vi "总磷总氮通讯.vi"() -> ()   [LabVIEW 2016, in "斯坦道总磷总氮.lvlib"]
uses:
  <vilib>/NI/Modbus Library/API/Wrapper/Create TCP Slave.vi
  <vilib>/Utility/config.llb/Write Key (Boolean).vi
  <vilib>/Utility/config.llb/Write Key (String).vi
  <vilib>/Plasmionique/MB Master/MB_Master/MB_Master.lvclass
  <vilib>/NI/Modbus Library/API/slave/Modbus Slave.lvclass
  <vilib>/Utility/config.llb/NI_LVConfig.lvlib
  <vilib>/Plasmionique/MB Master/MB Master.lvlib
  <vilib>/NI/Modbus Library/API/Wrapper/API Main.lvlib
panel:
  out "总氮测量数据区":u16[](array[numeric])
  out "总氮状态告警区":u16[](array[numeric])
  out "总磷状态告警区":u16[](array[numeric])
  out "总磷测量数据区":u16[](array[numeric])
  out "序列号":string
  out "状态告警区":T1 {"告警代码" items=["无告警", "缺试剂告警", "缺水样告警", "缺蒸馏水告警", "缺标液告警", "仪表漏液告警", "标定异常告警", "超量程告警", "加热异常", "低试剂预警", "超上限告警", "超下限告警", "仪表内部其他异常", "滴定异常告警", "电极异常告警", "量程切换告警", "参数设置告警", "PH电极电位异常", "电导率电极异常", "浊度光度异常", "溶解氧电极异常", "溶解氧光强异常", "温度异常告警", "PH异常告警", "溶解氧异常告警", "电导率异常告警", "浊度异常告警", "叶绿素异常告警", "藻密度异常告警", "蓝绿藻异常告警", "ORP异常告警", "氨氮异常告警", "清洁刷异常告警", "SD卡异常告警", "蓝牙异常告警", "Wifi异常告警", "流程异常告警"]; "故障代码" items=["无故障", "电机故障", "温度故障", "通讯故障", "滴定故障"]}
  out "测量数据区":T2 {"单位" items=["ug/L", "mg/L", "ppm", "mg/m3", "cm", "ppb", "ug/m3", "%", "nmol/mol", "umol/mol", "MPN/L", "MPN/100ml", "ng/m3", "NTU", "无量纲", "ms/cm", "us/cm", "℃", "mV", "万个/L"]}
  out "status":bool
  out "关键参数区":T3
  in  "读关键参数区":bool
  in  "读状态告警区":bool
  in  "读测量数据区":bool
  in  "站号":u16(ring) items=["总磷"=1, "氨氮"=3]
  in  "停止":bool
  in  "启动":bool
  in  "控制命令":u16(ring) items=["启动测量"=1, "标样核查"=2, "零点核查"=3, "跨度核查"=4, "空白测试"=5, "平行样测试"=6, "加标回收"=7, "空白校准"=8, "标样校准"=9, "初始化（清洗）"=10, "停止测试"=11, "仪器重启"=12, "校时"=13, "模式设置"=14, "测量间隔设置"=15]
  in  "控制命令参数":u16[](array[numeric]) format="%04xH"
  in  "VISA Resource":refnum<visa-resource-name>
  in  "启用模块":bool
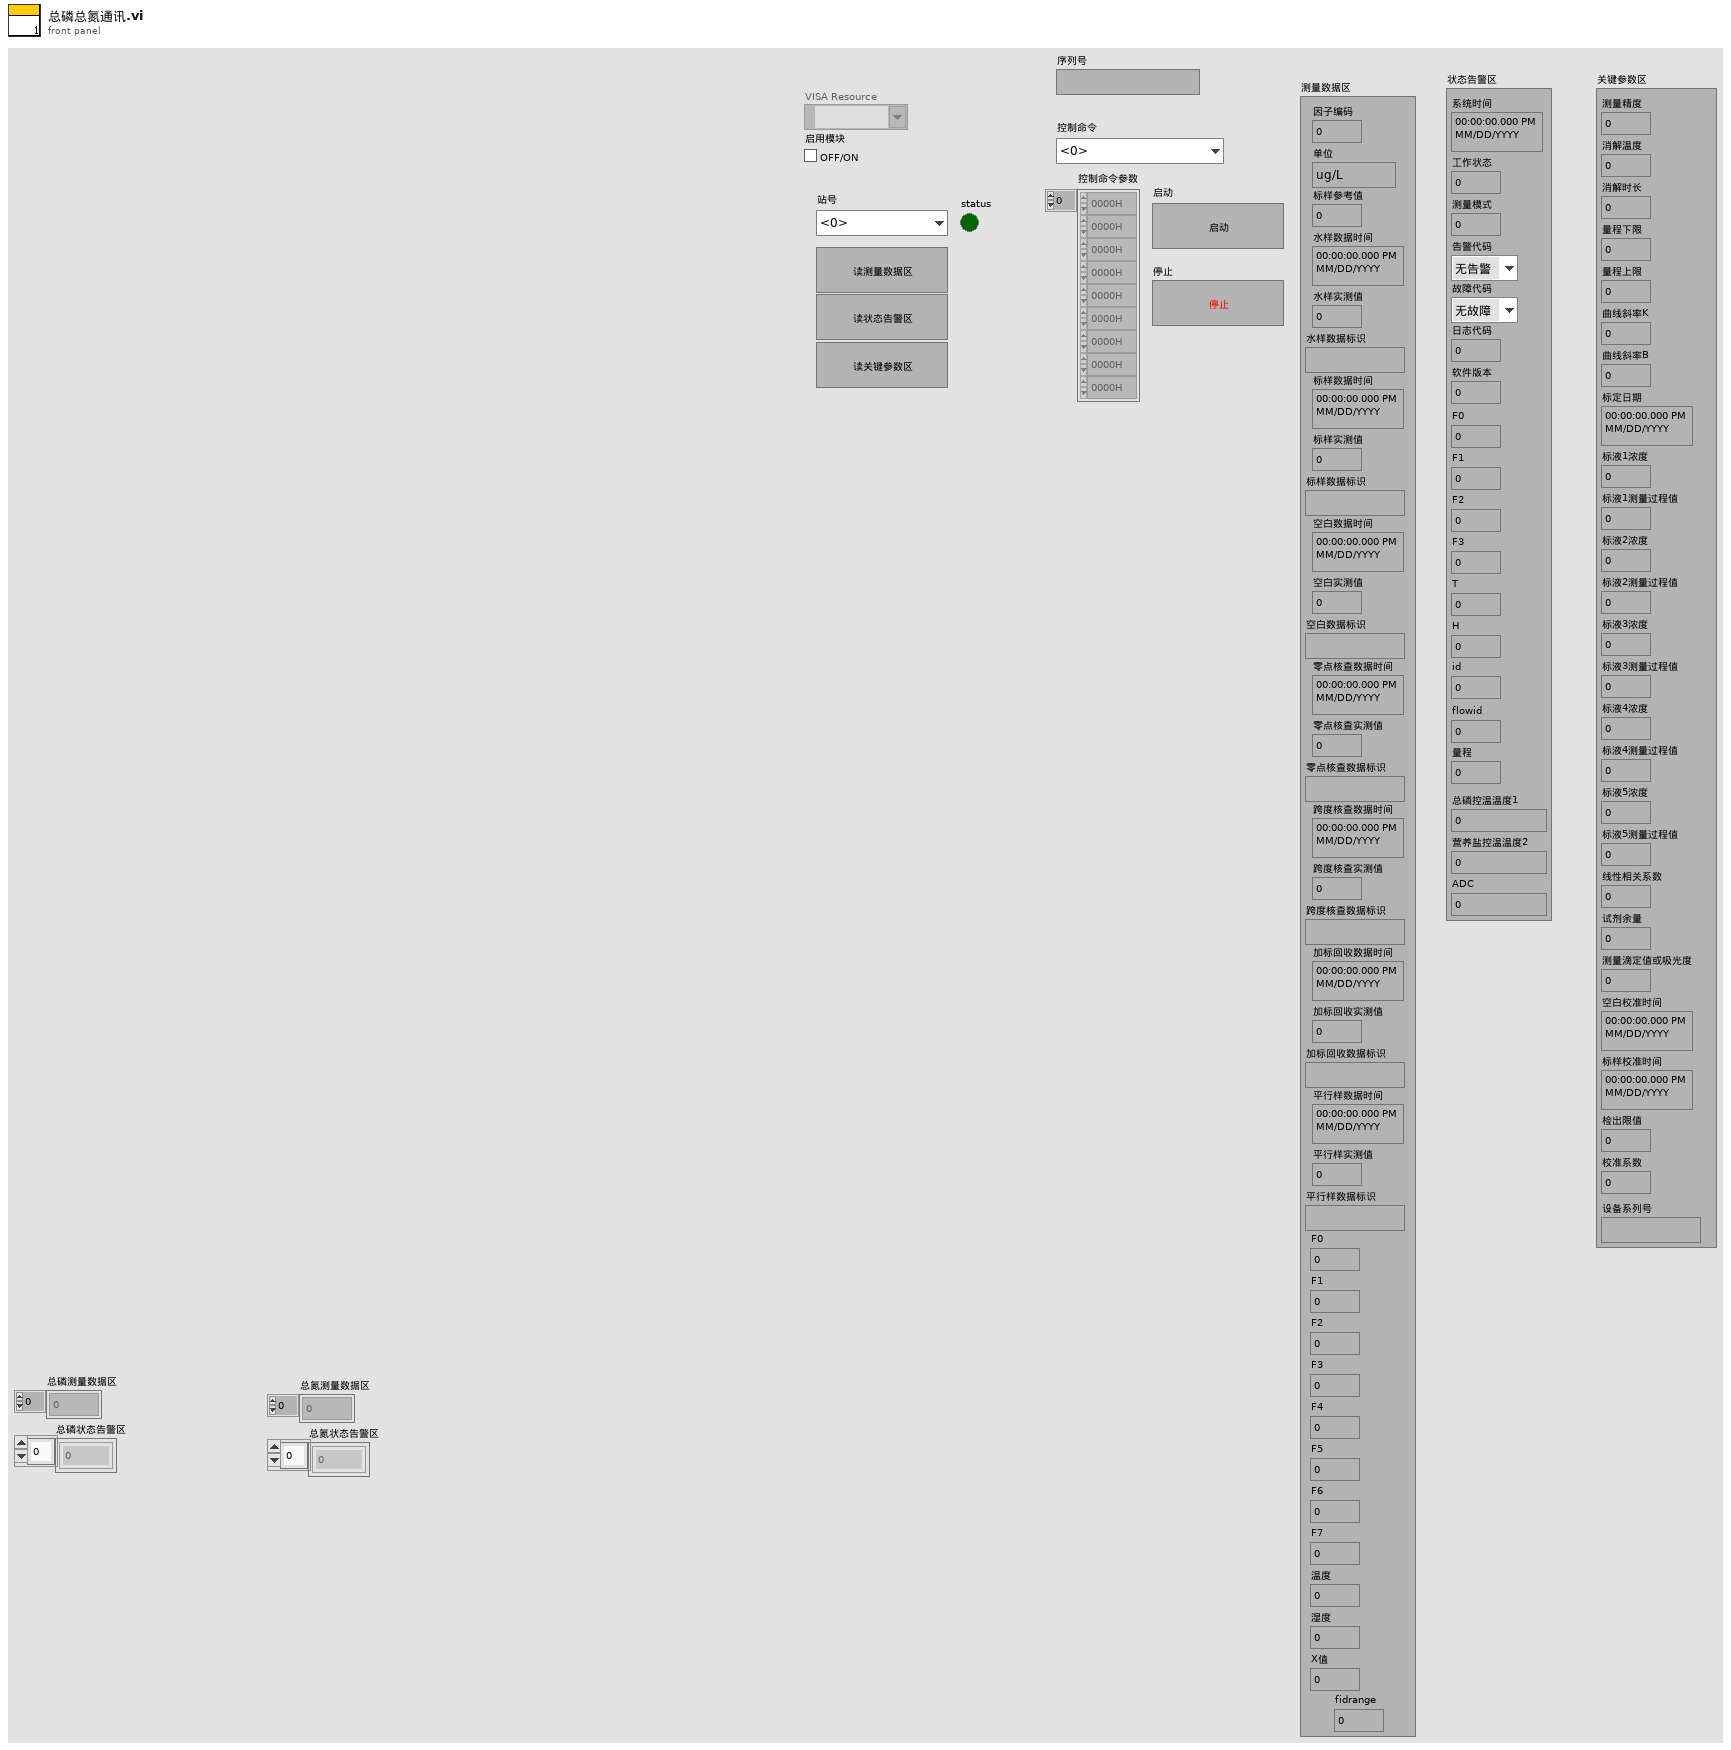
[diagram p1: front panel]
types:
  T1 = cluster{"系统时间":timestamp, "工作状态":u16, "测量模式":u16, "告警代码":u16, "故障代码":u16, "日志代码":u16, "软件版本":u16, "F0":sgl, "F1":sgl, "F2":sgl, "F3":sgl, "T":sgl, "H":sgl, "id":u16, "flowid":u16, "量程":u16, "总磷控温温度1":sgl, "营养盐控温温度2":sgl, "ADC":sgl}
  T2 = cluster{"因子编码":u32, "单位":u16, "标样参考值":sgl, "水样数据时间":timestamp, "水样实测值":sgl, "水样数据标识":string, "标样数据时间":timestamp, "标样实测值":sgl, "标样数据标识":string, "空白数据时间":timestamp, "空白实测值":sgl, "空白数据标识":string, "零点核查数据时间":timestamp, "零点核查实测值":sgl, "零点核查数据标识":string, "跨度核查数据时间":timestamp, "跨度核查实测值":sgl, "跨度核查数据标识":string, "加标回收数据时间":timestamp, "加标回收实测值":sgl, "加标回收数据标识":string, "平行样数据时间":timestamp, "平行样实测值":sgl, "平行样数据标识":string, "F0":sgl, "F1":sgl, "F2":sgl, "F3":sgl, "F4":sgl, "F5":sgl, "F6":sgl, "F7":sgl, "温度":sgl, "湿度":sgl, "X值":sgl, "fidrange":u16}
  T3 = cluster{"测量精度":u16, "消解温度":u16, "消解时长":u16, "量程下限":sgl, "量程上限":sgl, "曲线斜率K":sgl, "曲线斜率B":sgl, "标定日期":timestamp, "标液1浓度":sgl, "标液1测量过程值":sgl, "标液2浓度":sgl, "标液2测量过程值":sgl, "标液3浓度":sgl, "标液3测量过程值":sgl, "标液4浓度":sgl, "标液4测量过程值":sgl, "标液5浓度":sgl, "标液5测量过程值":sgl, "线性相关系数":sgl, "试剂余量":u32, "测量滴定值或吸光度":sgl, "空白校准时间":timestamp, "标样校准时间":timestamp, "检出限值":sgl, "校准系数":sgl, "设备系列号":string}
  T4 = typedef "NI_LVConfig.lvlib/Config Data RefNum.ctl" = refnum<k1>
  T5 = enum8{"Enabled", "Disabled", "Disabled and Grayed Out"}
  T6 = cluster{"系统时间":timestamp, "工作状态":enum16{"空闲", "水样测试", "标样核查", "零点核查", "跨度核查", "空白测试", "平行样测试", "加标回收", "空白校准", "标样校准", "初始化（清洗）"}, "测量模式":enum16{"待机", "连续模式", "周期模式", "定点模式", "受控模式", "手动模式"}, "告警代码":u16, "故障代码":u16, "日志代码":u16, "软件版本":u16, "F0":sgl, "F1":sgl, "F2":sgl, "F3":sgl, "T":sgl, "H":sgl, "id":u16, "flowid":u16, "量程":u16, "总磷控温温度1":sgl, "营养盐控温温度2":sgl, "ADC":sgl}
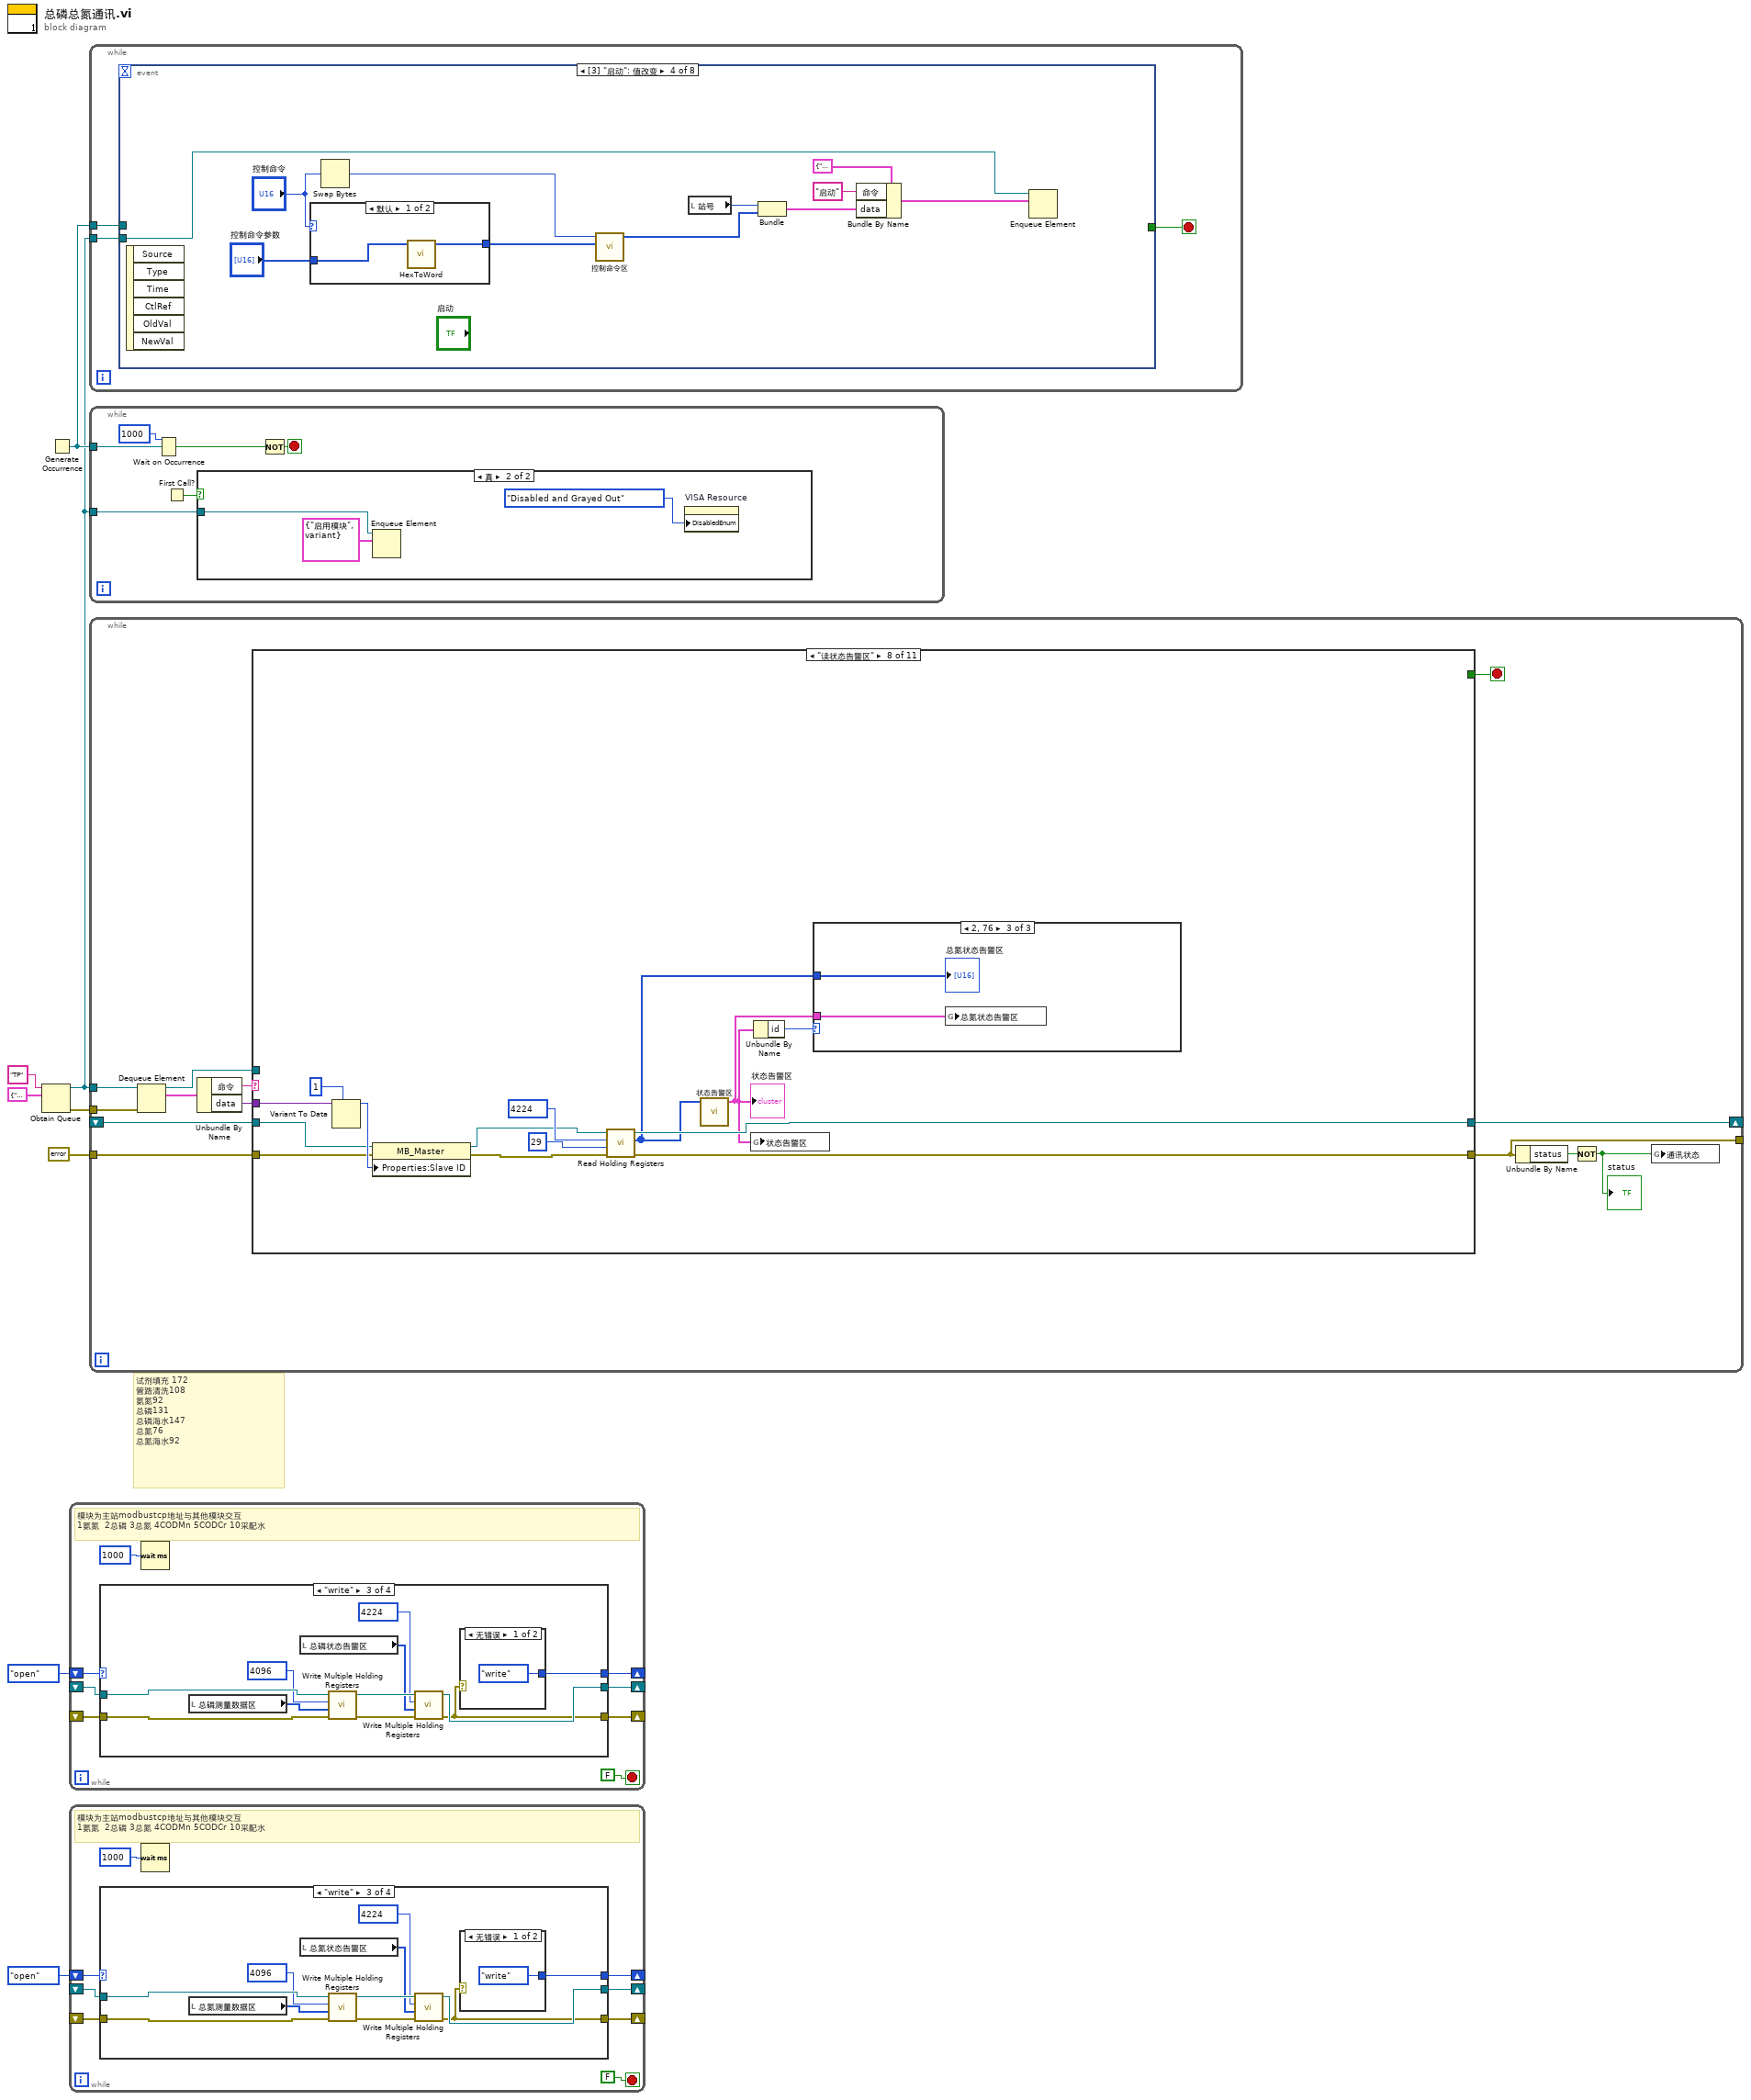
[diagram p0: block diagram]
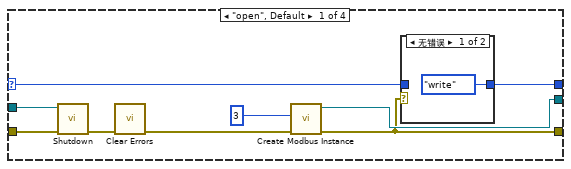
[diagram p2: hidden frame]
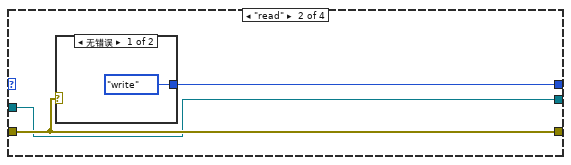
[diagram p4: hidden frame]
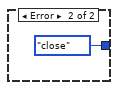
[diagram p5: hidden frame]
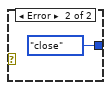
[diagram p6: hidden frame]
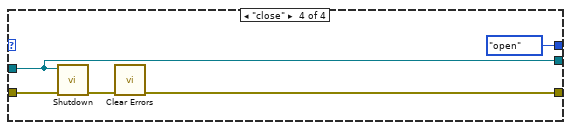
[diagram p7: hidden frame]
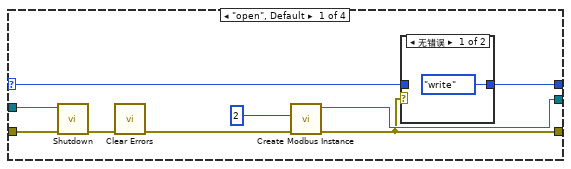
[diagram p8: hidden frame]
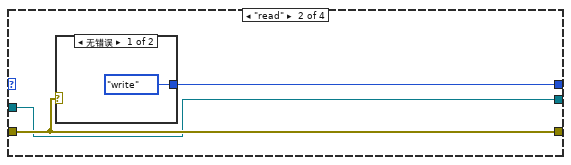
[diagram p10: hidden frame]
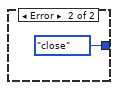
[diagram p11: hidden frame]
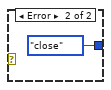
[diagram p12: hidden frame]
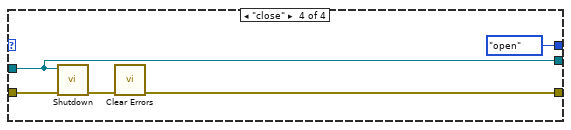
[diagram p13: hidden frame]
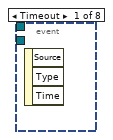
[diagram p15: hidden frame]
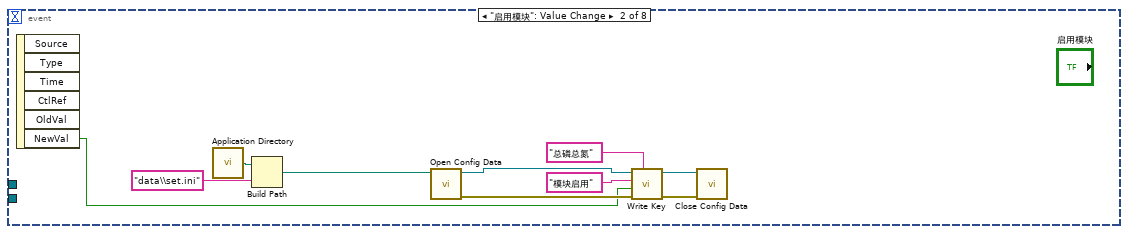
[diagram p16: hidden frame]
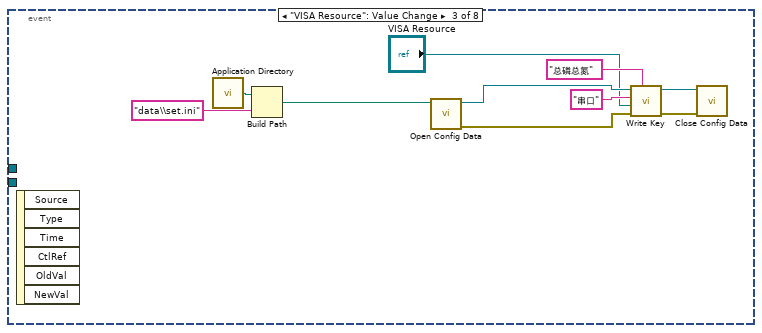
[diagram p17: hidden frame]
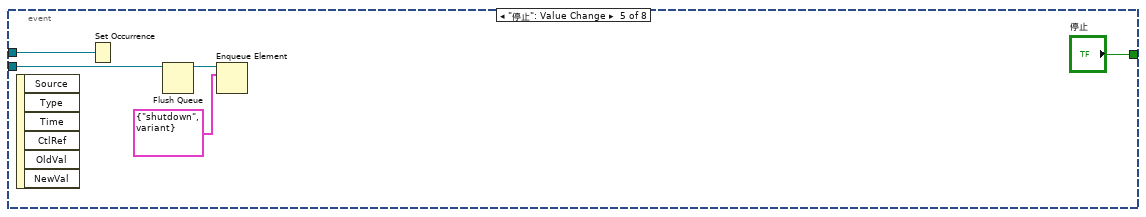
[diagram p19: hidden frame]
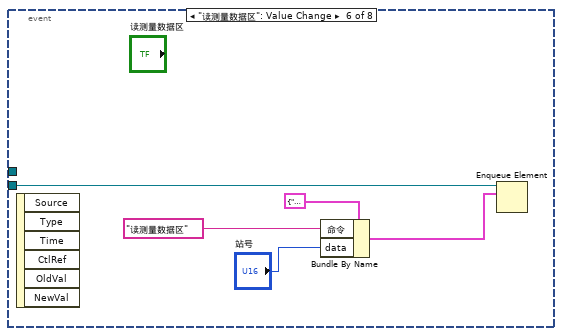
[diagram p20: hidden frame]
diagram:
  # "试剂填充 172 \n管路清洗108\n氨氮92\n总磷131\n总磷海水147\n总氮76\n总氮海水92"
  n1 = Obtain Queue(name (unnamed)="TP" ("名称（未命名）"), element data type=cluster{"命令":string, "data":variant} {"命令"="", "data"=variant}) -> (queue out=w3:refnum<queue>, error out=w6:errorcluster)  [unwired: 3 in, 1 out]
  n2 = Generate Occurrence() -> (w4:refnum<k4>)
  n3 = while {
    shift-right: [w14] -> _
    shift-left: _ -> [w16]
    shift-right: [w13] -> _
    shift-left: _ -> [w15]
    shift-right: [w10] -> _
    shift-left: enum16{"open", "read", "write", "close"}."open" -> [w11]
    stop <- FALSE stop-if-true
    # "模块为主站modbustcp地址与其他模块交互\n1氨氮  2总磷 3总氮 4CODMn 5CODCr 10采配水"
    n4 = case shown="\"write\"" w11 {
      selector: w11 -> [w25 _ _ _]
      tunnel: w16 -> [w19 w28 w42 w48]
      tunnel: w15 -> [w18 w29 w41 w47]
      tunnel: [w22 w28 w37 w48] -> w14
      tunnel: [w21 w29 w36 w50] -> w13
      tunnel: [w24 w30 w43 enum16{"open", "read", "write", "close"}."open"] -> w10
      frame "open", Default {
        n5 = call-dynamic "Shutdown.vi"("error in"=w18, "Modbus slave in"=w19) -> ("error out"=w17:errorcluster)  [unwired: 9 in]
        n6 = call <vilib>:"Clear Errors.vi"("error in (no error)"=w17) -> ("error out"=w20:errorcluster)  [unwired: 5 in, 1 out]
        n7 = call-poly <vilib>:"Create Modbus Instance.vi"("error in"=w20, "port (502)"=u16 2) -> ("error out"=w21:errorcluster, "TCP slave instance"=w22:refnum<class "Modbus Slave.lvclass">)  [unwired: 8 in]
        n8 = case shown="无错误" w21 {
          tunnel: w25 -> [_ w27]
          tunnel: [enum16{"open", "read", "write", "close"}."write" w27] -> w24
          frame No Error {
          }
          frame Error {
          }
        }
      }
      frame "read" {
        n9 = case shown="无错误" w29 {
          tunnel: [enum16{"open", "read", "write", "close"}."write" enum16{"open", "read", "write", "close"}."close"] -> w30
          frame No Error {
          }
          frame Error {
          }
        }
      }
      frame "write" {
        n10 = local read "总磷测量数据区"() -> (w35:u16[])
        n11 = local read "总磷状态告警区"() -> (w33:u16[])
        n12 = call-dynamic "Write Multiple Holding Registers.vi"("error in"=w41, "registers to write"=w35, "starting address"=u16 4096, "Modbus slave in"=w42) -> ("error out"=w38:errorcluster, "Modbus slave out"=w39:refnum<class "Modbus Slave.lvclass">)  [unwired: 6 in]
        n13 = call-dynamic "Write Multiple Holding Registers.vi"("error in"=w38, "registers to write"=w33, "starting address"=u16 4224, "Modbus slave in"=w39) -> ("error out"=w36:errorcluster, "Modbus slave out"=w37:refnum<class "Modbus Slave.lvclass">)  [unwired: 6 in]
        n14 = case shown="无错误" w36 {
          tunnel: [enum16{"open", "read", "write", "close"}."write" enum16{"open", "read", "write", "close"}."close"] -> w43
          frame No Error {
          }
          frame Error {
          }
        }
      }
      frame "close" {
        n15 = call-dynamic "Shutdown.vi"("error in"=w47, "Modbus slave in"=w48) -> ("error out"=w46:errorcluster)  [unwired: 9 in]
        n16 = call <vilib>:"Clear Errors.vi"("error in (no error)"=w46) -> ("error out"=w50:errorcluster)  [unwired: 5 in, 1 out]
      }
    }
    n17 = Wait (ms)(milliseconds to wait=u32 1000 ("等待时间（毫秒）")) -> ()  [unwired: 1 out]
  }
  n18 = while {
    shift-right: [w56] -> _
    shift-left: _ -> [w58]
    shift-right: [w55] -> _
    shift-left: _ -> [w57]
    shift-right: [w52] -> _
    shift-left: enum16{"open", "read", "write", "close"}."open" -> [w53]
    stop <- FALSE stop-if-true
    # "模块为主站modbustcp地址与其他模块交互\n1氨氮  2总磷 3总氮 4CODMn 5CODCr 10采配水"
    n19 = case shown="\"write\"" w53 {
      selector: w53 -> [w67 _ _ _]
      tunnel: w58 -> [w61 w70 w84 w90]
      tunnel: w57 -> [w60 w71 w83 w89]
      tunnel: [w64 w70 w79 w90] -> w56
      tunnel: [w63 w71 w78 w92] -> w55
      tunnel: [w66 w72 w85 enum16{"open", "read", "write", "close"}."open"] -> w52
      frame "open", Default {
        n20 = call-dynamic "Shutdown.vi"("error in"=w60, "Modbus slave in"=w61) -> ("error out"=w59:errorcluster)  [unwired: 9 in]
        n21 = call <vilib>:"Clear Errors.vi"("error in (no error)"=w59) -> ("error out"=w62:errorcluster)  [unwired: 5 in, 1 out]
        n22 = call-poly <vilib>:"Create Modbus Instance.vi"("error in"=w62, "port (502)"=u16 3) -> ("error out"=w63:errorcluster, "TCP slave instance"=w64:refnum<class "Modbus Slave.lvclass">)  [unwired: 8 in]
        n23 = case shown="无错误" w63 {
          tunnel: w67 -> [_ w69]
          tunnel: [enum16{"open", "read", "write", "close"}."write" w69] -> w66
          frame No Error {
          }
          frame Error {
          }
        }
      }
      frame "read" {
        n24 = case shown="无错误" w71 {
          tunnel: [enum16{"open", "read", "write", "close"}."write" enum16{"open", "read", "write", "close"}."close"] -> w72
          frame No Error {
          }
          frame Error {
          }
        }
      }
      frame "write" {
        n25 = local read "总氮测量数据区"() -> (w77:u16[])
        n26 = local read "总氮状态告警区"() -> (w75:u16[])
        n27 = call-dynamic "Write Multiple Holding Registers.vi"("error in"=w83, "registers to write"=w77, "starting address"=u16 4096, "Modbus slave in"=w84) -> ("error out"=w80:errorcluster, "Modbus slave out"=w81:refnum<class "Modbus Slave.lvclass">)  [unwired: 6 in]
        n28 = call-dynamic "Write Multiple Holding Registers.vi"("error in"=w80, "registers to write"=w75, "starting address"=u16 4224, "Modbus slave in"=w81) -> ("error out"=w78:errorcluster, "Modbus slave out"=w79:refnum<class "Modbus Slave.lvclass">)  [unwired: 6 in]
        n29 = case shown="无错误" w78 {
          tunnel: [enum16{"open", "read", "write", "close"}."write" enum16{"open", "read", "write", "close"}."close"] -> w85
          frame No Error {
          }
          frame Error {
          }
        }
      }
      frame "close" {
        n30 = call-dynamic "Shutdown.vi"("error in"=w89, "Modbus slave in"=w90) -> ("error out"=w88:errorcluster)  [unwired: 9 in]
        n31 = call <vilib>:"Clear Errors.vi"("error in (no error)"=w88) -> ("error out"=w92:errorcluster)  [unwired: 5 in, 1 out]
      }
    }
    n32 = Wait (ms)(milliseconds to wait=u32 1000 ("等待时间（毫秒）")) -> ()  [unwired: 1 out]
  }
  n33 = while {
    tunnel: w3 -> [w95]
    tunnel: w4 -> [w93]
    stop <- w94 stop-if-true
    n34 = event shown="[3] \"启动\": 值改变" {
      selector: _ -> [_ _ _ _ _ _ _ _]
      dyn-events: _ -> [_ _ _ _ _ _ _ _]
      timeout: _ -> [_ _ _ _ _ _ _ _]
      tunnel: w95 -> [_ _ _ w126 w133 w139 w144 w149]
      tunnel: [_ _ _ _ "停止" _ _ _] -> w94
      tunnel: w93 -> [_ _ _ _ w130 _ _ _]
      event Timeout {
        n35 = event-data() -> ()  [unwired: 1 in, 3 out]
      }
      event "启用模块": Value Change {
        n36 = event-data() -> ("NewVal"=w96:bool)  [unwired: 1 in, 5 out]
        n37 = call <vilib>:"Application Directory.vi"() -> ("Application Directory"=w98:path)
        n38 = Build Path(base path=w98, name or relative path="data\\set.ini" ("名称或相对路径")) -> (appended path=w99:path)
        n39 = call <vilib>:"Open Config Data.vi"("configuration file path"=w99) -> ("error out"=w105:errorcluster, "refnum"=w104:T4)  [unwired: 8 in, 1 out]
        n40 = call-poly <vilib>:"Write Key.vi"("section"="总磷总氮", "error in (no error)"=w105, "value"=w96, "key"="模块启用", "refnum"=w104) -> ("error out"=w101:errorcluster, "refnum out"=w97:T4)  [unwired: 4 in, 1 out]
        n41 = call <vilib>:"Close Config Data.vi"("error in (no error)"=w101, "refnum"=w97) -> ()  [unwired: 8 in, 2 out]
      }
      event "VISA Resource": Value Change {
        n42 = event-data() -> ()  [unwired: 1 in, 6 out]
        n43 = call <vilib>:"Application Directory.vi"() -> ("Application Directory"=w108:path)
        n44 = Build Path(base path=w108, name or relative path="data\\set.ini" ("名称或相对路径")) -> (appended path=w109:path)
        n45 = call <vilib>:"Open Config Data.vi"("configuration file path"=w109) -> ("error out"=w115:errorcluster, "refnum"=w114:T4)  [unwired: 8 in, 1 out]
        n46 = call-poly <vilib>:"Write Key.vi"("section"="总磷总氮", "error in (no error)"=w115, "value"="VISA Resource", "key"="串口", "refnum"=w114) -> ("error out"=w111:errorcluster, "refnum out"=w107:T4)  [unwired: 4 in, 1 out]
        n47 = call <vilib>:"Close Config Data.vi"("error in (no error)"=w111, "refnum"=w107) -> ()  [unwired: 8 in, 2 out]
      }
      event "启动": Value Change {
        n48 = event-data() -> ()  [unwired: 1 in, 6 out]
        n49 = case shown="默认" "控制命令" {
          tunnel: "控制命令参数" -> [w128 w129]
          tunnel: [w127 w129] -> w116
          frame Default {
            n50 = call "HexToWord.vi"("数组"=w128) -> ("WORD"=w127:u16[])  [unwired: 10 in]
          }
          frame 13 {
          }
        }
        n51 = Swap Bytes(anything="控制命令") -> (byte swapped=w119:u16)
        n52 = call "控制命令区.vi"("控制命令参数"=w116, "控制命令"=w119) -> ("控制命令"=w122:u16[])  [unwired: 9 in]
        n53 = local read "站号"() -> (w121:u16)
        n54 = Bundle("站号"=w121, "控制命令"=w122) -> (w120:cluster{"站号":u16, "控制命令":u16[]})  [unwired: 1 in]
        n55 = Bundle By Name(cluster=cluster{"命令":string, "data":variant} {"命令"="", "data"=variant} ("元素"), "命令"="启动", "data"=w120) -> (w124:cluster{"命令":string, "data":variant})
        n56 = Enqueue Element(queue=w126, element=w124) -> ()  [unwired: 2 in, 3 out]
      }
      event "停止": Value Change {
        n57 = event-data() -> ()  [unwired: 1 in, 6 out]
        n58 = Set Occurrence(w130) -> ()
        n59 = Flush Queue(queue=w133) -> (queue out=w132:refnum<queue>)  [unwired: 1 in, 2 out]
        n60 = Enqueue Element(queue=w132, element=cluster{"命令":string, "data":variant} {"命令"="shutdown", "data"=variant} ("元素")) -> ()  [unwired: 2 in, 3 out]
      }
      event "读测量数据区": Value Change {
        n61 = event-data() -> ()  [unwired: 1 in, 6 out]
        n62 = Bundle By Name(cluster=cluster{"命令":string, "data":variant} {"命令"="", "data"=variant} ("元素"), "命令"="读测量数据区", "data"="站号") -> (w137:cluster{"命令":string, "data":variant})
        n63 = Enqueue Element(queue=w139, element=w137) -> ()  [unwired: 2 in, 3 out]
      }
      event "读状态告警区": Value Change {
        n64 = event-data() -> ()  [unwired: 1 in, 6 out]
        n65 = local read "站号"() -> (w140:u16)
        n66 = Bundle By Name(cluster=cluster{"命令":string, "data":variant} {"命令"="", "data"=variant} ("元素"), "命令"="读状态告警区", "data"=w140) -> (w142:cluster{"命令":string, "data":variant})
        n67 = Enqueue Element(queue=w144, element=w142) -> ()  [unwired: 2 in, 3 out]
      }
      event "读关键参数区": Value Change {
        n68 = event-data() -> ()  [unwired: 1 in, 6 out]
        n69 = local read "站号"() -> (w145:u16)
        n70 = Bundle By Name(cluster=cluster{"命令":string, "data":variant} {"命令"="", "data"=variant} ("元素"), "命令"="读关键参数区", "data"=w145) -> (w147:cluster{"命令":string, "data":variant})
        n71 = Enqueue Element(queue=w149, element=w147) -> ()  [unwired: 2 in, 3 out]
      }
    }
  }
  n72 = while {
    tunnel: w4 -> [w155]
    tunnel: w3 -> [w151]
    stop <- w152 stop-if-true
    n73 = Wait on Occurrence(2:w155, 3:1000 ("毫秒超时(-1)")) -> (0:w153:bool)  [unwired: 1 in]
    n74 = First Call?() -> (First Call?: T/F=w150:bool)
    n75 = case shown="真" w150 {
      tunnel: w151 -> [_ w157]
      frame False {
      }
      frame True {
        n76 = Enqueue Element(queue=w157, element=cluster{"命令":string, "data":variant} {"命令"="启用模块", "data"=variant} ("元素")) -> ()  [unwired: 2 in, 3 out]
        n77 = property on="VISA Resource" class="VISAName"("DisabledEnum"=T5."Disabled and Grayed Out" ("禁用")) -> ()  [unwired: 2 in, 2 out]
      }
    }
    n78 = Not(x=w153) -> (.not. x?=w152:bool)
  }
  n79 = while {
    tunnel: w3 -> [w171]
    tunnel: w6 -> [w170]
    shift-right: [w168] -> _
    shift-left: _ -> [w167]
    tunnel: errorcluster {"status"=FALSE, "code"=0, "source"=""} ("error out") -> [w166]
    tunnel: [w161] -> _
    stop <- w169 stop-if-true
    n80 = Dequeue Element(queue=w171, error in (no error)=w170) -> (queue out=w162:refnum<queue>, element=w164:cluster{"命令":string, "data":variant})  [unwired: 1 in, 2 out]
    n81 = Unbundle By Name(w164) -> ("命令"=w165:string, "data"=w163:variant)
    n82 = case shown="\"读状态告警区\"" w165 {
      tunnel: w163 -> [_ _ _ w190 w201 w218 w228 w261 w279 w293 _]
      tunnel: w162 -> [_ _ _ _ _ _ _ _ _ _ w306]
      tunnel: [_ _ _ _ _ _ _ _ _ _ TRUE] -> w169
      tunnel: [w172 w174 w177 w193 w204 w220 w232 w270 w286 w300 w302] -> w168
      tunnel: [w173 w175 w178 w192 w203 w219 w233 w260 w287 w301 w303] -> w161
      tunnel: w167 -> [w172 _ w177 w189 w200 w217 w227 w264 w282 w296 w302]
      tunnel: w166 -> [w173 _ w180 w186 w197 w214 w225 w265 w283 w297 w304]
      frame Default {
      }
      frame "启用模块" {
        n83 = call "总磷总氮MB_api.vi"("STEP"=enum16{"open", "read", "write", "close"}."open") -> ("error out"=w175:errorcluster, "MB session out"=w174:refnum<class "MB_Master.lvclass">)  [unwired: 8 in, 1 out]
        n84 = global write "VAR总磷总氮全局变量.vi" "MB session in"(w174) -> ()
      }
      frame "停用模块" {
        n85 = call-dynamic "Close Session.vi"("error in (no error)"=w180, "MB session in"=w177) -> ("error out"=w179:errorcluster)  [unwired: 9 in]
        n86 = call <vilib>:"Clear Errors.vi"("error in (no error)"=w179) -> ("error out"=w178:errorcluster)  [unwired: 5 in, 1 out]
      }
      frame "启动" {
        n87 = Variant To Data(type=cluster{"站号":u16, "控制命令":u16[]} {"站号"=0, "控制命令"=[]} ("输出簇"), Variant=w190) -> (data=w184:cluster{"站号":u16, "控制命令":u16[]})  [unwired: 1 in, 1 out]
        n88 = Unbundle By Name(w184) -> ("站号"=w183:u16, "控制命令"=w181:u16[])
        n89 = property class="MB_Master"(reference=w189, error in=w186, "Properties:Slave ID"=w183) -> (reference out=w188:refnum<class "MB_Master.lvclass">, error out=w187:errorcluster)
        n90 = Index Array(array=w181) -> (element=w182:u16)  [unwired: 1 in]
        n91 = global write "VAR总磷总氮全局变量.vi" "控制命令"(w182) -> ()
        n92 = call <vilib>:"Write Multiple Registers.vi"("error in (no error)"=w187, "values"=w181, "starting address"=u16 4608, "MB session in"=w188) -> ("error out"=w192:errorcluster, "MB session out"=w193:refnum<class "MB_Master.lvclass">)  [unwired: 6 in]
      }
      frame "盲样测试" {
        n93 = Variant To Data(type=0, Variant=w201) -> (data=w194:i32)  [unwired: 1 in, 1 out]
        n94 = case shown="默认" w194 {
          tunnel: [u16[] [] ("values") u16[] [33539, 0] ("values") u16[] [23555, 0] ("values")] -> w196
          frame Default {
          }
          frame 1 {
            # "总磷盲样测试命令"
          }
          frame 3 {
            # "氨氮盲样测试"
          }
        }
        n95 = property class="MB_Master"(reference=w200, error in=w197, "Properties:Slave ID"=w194) -> (reference out=w199:refnum<class "MB_Master.lvclass">, error out=w198:errorcluster)
        n96 = call <vilib>:"Write Multiple Registers.vi"("error in (no error)"=w198, "values"=w196, "starting address"=u16 24592, "MB session in"=w199) -> ("error out"=w203:errorcluster, "MB session out"=w204:refnum<class "MB_Master.lvclass">)  [unwired: 6 in]
      }
      frame "debug" {
        n97 = Variant To Data(type=cluster{"站号":u16, "控制命令":u16[]} {"站号"=0, "控制命令"=[]} ("输出簇"), Variant=w218) -> (data=w212:cluster{"站号":u16, "控制命令":u16[]})  [unwired: 1 in, 1 out]
        n98 = Unbundle By Name(w212) -> ("站号"=w211:u16, "控制命令"=w209:u16[])
        n99 = property class="MB_Master"(reference=w217, error in=w214, "Properties:Slave ID"=w211) -> (reference out=w216:refnum<class "MB_Master.lvclass">, error out=w215:errorcluster)
        n100 = Index Array(array=w209) -> (element=w210:u16)  [unwired: 1 in]
        n101 = global write "VAR总磷总氮全局变量.vi" "控制命令"(w210) -> ()
        n102 = call <vilib>:"Write Multiple Registers.vi"("error in (no error)"=w215, "values"=w209, "starting address"=u16 24594, "MB session in"=w216) -> ("error out"=w219:errorcluster, "MB session out"=w220:refnum<class "MB_Master.lvclass">)  [unwired: 6 in]
      }
      frame "读测量数据区" {
        n103 = Variant To Data(type=u8 1 ("Slave ID"), Variant=w228) -> (data=w223:u8)  [unwired: 1 in, 1 out]
        n104 = property class="MB_Master"(reference=w227, error in=w225, "Properties:Slave ID"=w223) -> (reference out=w226:refnum<class "MB_Master.lvclass">, error out=w224:errorcluster)
        n105 = call <vilib>:"Read Holding Registers.vi"("error in (no error)"=w224, "quantity"=u16 105, "starting address"=u16 4096, "MB session in"=w226) -> ("error out"=w233:errorcluster, "Registers"=w221:u16[], "MB session out"=w232:refnum<class "MB_Master.lvclass">)  [unwired: 5 in]
        n106 = call "测量数据区.vi"("数组"=w221) -> ("测量数据区"=w222:T2)  [unwired: 10 in]
        "测量数据区" <- w222
        n107 = global write "VAR总磷总氮全局变量.vi" "测量数据区"(w222) -> ()
        n108 = case shown="1" w223 {
          tunnel: w222 -> [_ w254 w256]
          tunnel: w221 -> [_ w235 w255]
          frame 0, Default {
          }
          frame 1 {
            w234 = 1.0 ("f")
            n109 = Unbundle By Name(w254) -> ("水样实测值"=w253:sgl, "标样实测值"=w251:sgl, "空白实测值"=w249:sgl, "零点核查实测值"=w247:sgl, "跨度核查实测值"=w245:sgl, "加标回收实测值"=w243:sgl, "平行样实测值"=w241:sgl)
            n110 = Multiply(x=w253, y=w234) -> (x*y=w252:dbl)
            n111 = Multiply(x=w251, y=w234) -> (x*y=w250:dbl)
            n112 = Multiply(x=w249, y=w234) -> (x*y=w248:dbl)
            n113 = Multiply(x=w247, y=w234) -> (x*y=w246:dbl)
            n114 = Multiply(x=w245, y=w234) -> (x*y=w244:dbl)
            n115 = Multiply(x=w243, y=w234) -> (x*y=w242:dbl)
            n116 = Multiply(x=w241, y=w234) -> (x*y=w240:dbl)
            n117 = global read "VAR总磷总氮全局变量.vi" "总氮测量数据区"() -> (w238:T2)
            n118 = global read "VAR总磷总氮全局变量.vi" "总磷测量数据区"() -> (w236:T2)
            n119 = Bundle By Name(cluster=w254, "水样实测值"=w252, "标样实测值"=w250, "空白实测值"=w248, "零点核查实测值"=w246, "跨度核查实测值"=w244, "加标回收实测值"=w242, "平行样实测值"=w240) -> (w239:T2)
            n120 = call "总磷数据时间处理.vi"("总磷修正数据输入"=w236, "总氮原始数据"=w238, "总磷原始数据"=w239) -> ("总磷修正数据输出"=w237:T2)  [unwired: 8 in]
            n121 = global write "VAR总磷总氮全局变量.vi" "总磷测量数据区"(w237) -> ()
            "总磷测量数据区" <- w235
          }
          frame 2 {
            n122 = global write "VAR总磷总氮全局变量.vi" "总氮测量数据区"(w256) -> ()
            "总氮测量数据区" <- w255
          }
        }
      }
      frame "读状态告警区" {
        n123 = Variant To Data(type=u8 1 ("Slave ID"), Variant=w261) -> (data=w266:u8)  [unwired: 1 in, 1 out]
        n124 = property class="MB_Master"(reference=w264, error in=w265, "Properties:Slave ID"=w266) -> (reference out=w263:refnum<class "MB_Master.lvclass">, error out=w262:errorcluster)
        n125 = call <vilib>:"Read Holding Registers.vi"("error in (no error)"=w262, "quantity"=u16 29, "starting address"=u16 4224, "MB session in"=w263) -> ("error out"=w260:errorcluster, "Registers"=w257:u16[], "MB session out"=w270:refnum<class "MB_Master.lvclass">)  [unwired: 5 in]
        n126 = call "状态告警区.vi"("数组"=w257) -> ("状态告警区"=w258:T6)  [unwired: 10 in]
        "状态告警区" <- w258
        n127 = global write "VAR总磷总氮全局变量.vi" "状态告警区"(w258) -> ()
        n128 = Unbundle By Name(w258) -> ("id"=w259:u16)
        n129 = case shown="2, 76" w259 {
          tunnel: w258 -> [_ w272 w274]
          tunnel: w257 -> [_ w271 w273]
          frame 0, Default {
          }
          frame 1, 131 {
            n130 = global write "VAR总磷总氮全局变量.vi" "总磷状态告警区"(w272) -> ()
            "总磷状态告警区" <- w271
          }
          frame 2, 76 {
            n131 = global write "VAR总磷总氮全局变量.vi" "总氮状态告警区"(w274) -> ()
            "总氮状态告警区" <- w273
          }
        }
      }
      frame "读关键参数区" {
        n132 = Variant To Data(type=u8 1 ("Slave ID"), Variant=w279) -> (data=w277:u8)  [unwired: 1 in, 1 out]
        n133 = property class="MB_Master"(reference=w282, error in=w283, "Properties:Slave ID"=w277) -> (reference out=w281:refnum<class "MB_Master.lvclass">, error out=w280:errorcluster)
        n134 = call <vilib>:"Read Holding Registers.vi"("error in (no error)"=w280, "quantity"=u16 19, "starting address"=u16 4256, "MB session in"=w281) -> ("error out"=w287:errorcluster, "Registers"=w276:u16[], "MB session out"=w286:refnum<class "MB_Master.lvclass">)  [unwired: 5 in]
        n135 = call "关键参数区.vi"("数组"=w276) -> ("关键参数区"=w275:T3)  [unwired: 10 in]
        "关键参数区" <- w275
        n136 = global write "VAR总磷总氮全局变量.vi" "关键参数区"(w275) -> ()
      }
      frame "读序列号" {
        n137 = Variant To Data(type=u8 1 ("Slave ID"), Variant=w293) -> (data=w291:u8)  [unwired: 1 in, 1 out]
        n138 = property class="MB_Master"(reference=w296, error in=w297, "Properties:Slave ID"=w291) -> (reference out=w295:refnum<class "MB_Master.lvclass">, error out=w294:errorcluster)
        n139 = call <vilib>:"Read Holding Registers.vi"("error in (no error)"=w294, "quantity"=u16 6, "starting address"=u16 4, "MB session in"=w295) -> ("error out"=w301:errorcluster, "Registers"=w290:u16[], "MB session out"=w300:refnum<class "MB_Master.lvclass">)  [unwired: 5 in]
        n140 = call "HexToString.vi"("数组"=w290) -> ("STRING"=w289:string[])  [unwired: 10 in]
        n141 = Index Array(array=w289) -> (element=w288:string)  [unwired: 1 in]
        "序列号" <- w288
        n142 = global write "VAR总磷总氮全局变量.vi" "序列号"(w288) -> ()
      }
      frame "shutdown" {
        n143 = call-dynamic "Close Session.vi"("error in (no error)"=w304, "MB session in"=w302) -> ("error out"=w303:errorcluster)  [unwired: 9 in]
        n144 = Flush Queue(queue=w306) -> (queue out=w305:refnum<queue>)  [unwired: 1 in, 2 out]
        n145 = Release Queue(queue=w305) -> ()  [unwired: 2 in, 3 out]
      }
    }
    n146 = Unbundle By Name(w161) -> ("status"=w160:bool)
    n147 = Not(x=w160) -> (.not. x?=w159:bool)
    "status" <- w159
    n148 = global write "VAR总磷总氮全局变量.vi" "通讯状态"(w159) -> ()
  }
